vi "FdxCmdRxModeControlCvi.vi"(8 "error in":errorcluster, 9 "RxModeControlIn":T1 {"DefaultCronoMode" items=["FDX_RX_DEFAULT_ENA_CNT", "FDX_RX_DEFAULT_MON_ENA_ALL", "FDX_RX_DEFAULT_MON_ENA_GOOD"]; "DefaultPayloadMode" items=["FDX_PAYLOAD_FULL", "FDX_PAYLOAD_IP_EXT", "FDX_PAYLOAD_IP", "FDX_PAYLOAD_MAC"]; "ReceiveMode" items=["FDX_RX_CHRONO", "FDX_RX_VL"]}, 11 "InstrumentHandle_port":u32) -> (0 "error out":errorcluster, 1 "GlbMonBufferSizeOut":u32, 3 "InstrumentHandle_port":u32)   [LabVIEW 2020, in "AIM664LV.lvlib"]
doc: "This function is used to configure the operational mode of the receive port."
uses:
  AIM664LV.lvlib
  AFDX_LibraryAdmin/FdxGlobalDllPath.vi
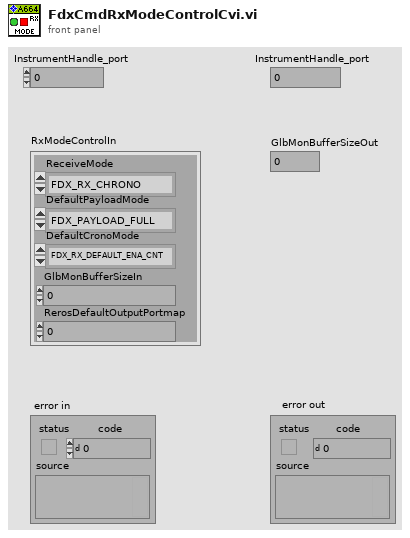
[diagram p1: front panel]
types:
  T1 = cluster{"ReceiveMode":u32, "DefaultPayloadMode":u32, "DefaultCronoMode":u32, "GlbMonBufferSizeIn":u32, "RerosDefaultOutputPortmap":u32}
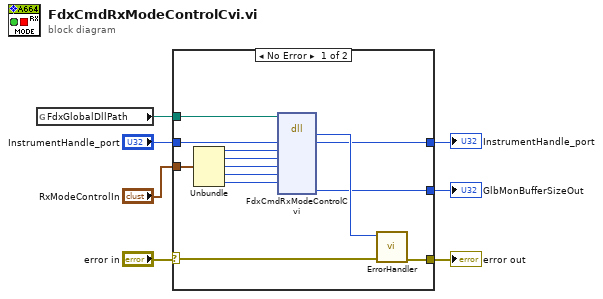
[diagram p0: block diagram]
diagram:
  n1 = global read "FdxGlobalDllPath.vi" "FdxGlobalDllPath"() -> (w5:path)
  n2 = case shown="No Error" "error in" {
    selector: "error in" -> [w19 w22]
    tunnel: [w20 w22] -> w7
    tunnel: w5 -> [w12 _]
    tunnel: "InstrumentHandle_port" -> [w11 w21]
    tunnel: [w10 w21] -> w3
    tunnel: "RxModeControlIn" -> [w9 _]
    tunnel: [w8 _] -> w1
    frame No Error {
      n3 = Unbundle(w9) -> ("ReceiveMode"=w17:u32, "DefaultPayloadMode"=w16:u32, "DefaultCronoMode"=w15:u32, "GlbMonBufferSizeIn"=w14:u32, "RerosDefaultOutputPortmap"=w13:u32)
      n4 = dll-call lib="aim_fdx.19.dll" fn="FdxCmdRxModeControlCvi"(path in=w12, "InstrumentHandle"=w11, "ReceiveMode"=w17, "DefaultPayloadMode"=w16, "DefaultCronoMode"=w15, "GlbMonBufferSizeIn"=w14, "RerosDefaultOutputPortmap"=w13) -> ("status"=w18:i32, "InstrumentHandle"=w10:u32, "GlbMonBufferSizeOut"=w8:u32)  [unwired: 7 in, 3 out]
      n5 = call "ErrorHandler.vi"("error in"=w19, "AIM Error"=w18) -> ("error out"=w20:errorcluster)  [unwired: 9 in]
    }
    frame Error {
    }
  }
  "error out" <- w7
  "InstrumentHandle_port" <- w3
  "GlbMonBufferSizeOut" <- w1
